vi "acquisition test fixed exposure 3.vi"() -> ()   [LabVIEW 2023]
uses:
  <vilib>/vision/driver/IMAQdx.llb/IMAQdx Attribute Type.ctl
  <vilib>/userDefined/High Color/IMAQdx.ctl
  <vilib>/vision/driver/IMAQdx.llb/IMAQdx Buffer Number Mode.ctl
  <vilib>/DAQmx/read.llb/DAQmx Read (Analog 1D Wfm NChan NSamp).vi
  <extravilib>/ChannelInstances/Tag-bool/Read With Abort.vi
  <extravilib>/ChannelInstances/Tag-bool/Write With Abort.vi
  <vilib>/DAQmx/create/channels.llb/DAQmx Create Channel (AI-Voltage-Basic).vi
  <vilib>/DAQmx/configure/timing.llb/DAQmx Timing (Sample Clock).vi
  <extravilib>/ChannelInstances/Tag-bool/Instantiate.vi
  <extravilib>/ChannelInstances/Tag-bool/EndpointRead.vi
  <extravilib>/ChannelInstances/Tag-bool/Endpoint.vi
  <vilib>/DAQmx/miscellaneous.llb/DAQmx Fill In Error Info.vi
  <extravilib>/ChannelInstances/Tag-bool.lvlib
  <vilib>/vision/driver/NI_Vision_Acquisition_Software.lvlib
  <resource>/objmgr/imaqdx.rc
panel:
  out "Maximum FrameRate":dbl
  out "Attribute Information":T2
  out "error out":errorcluster
  out "Sensor Readout Time":dbl
  out "Attribute Information Array 2":T3(array[cluster])
  out "Images Missed":u32
  out "Images Behind":i32
  out "Processed Frames per Second":dbl
  out "Acquired Frames per Second":dbl
  out "Image":T4(plugin-control)
  out "Waveform Chart":waveform(dbl)[](graph)
  in  "stop":bool
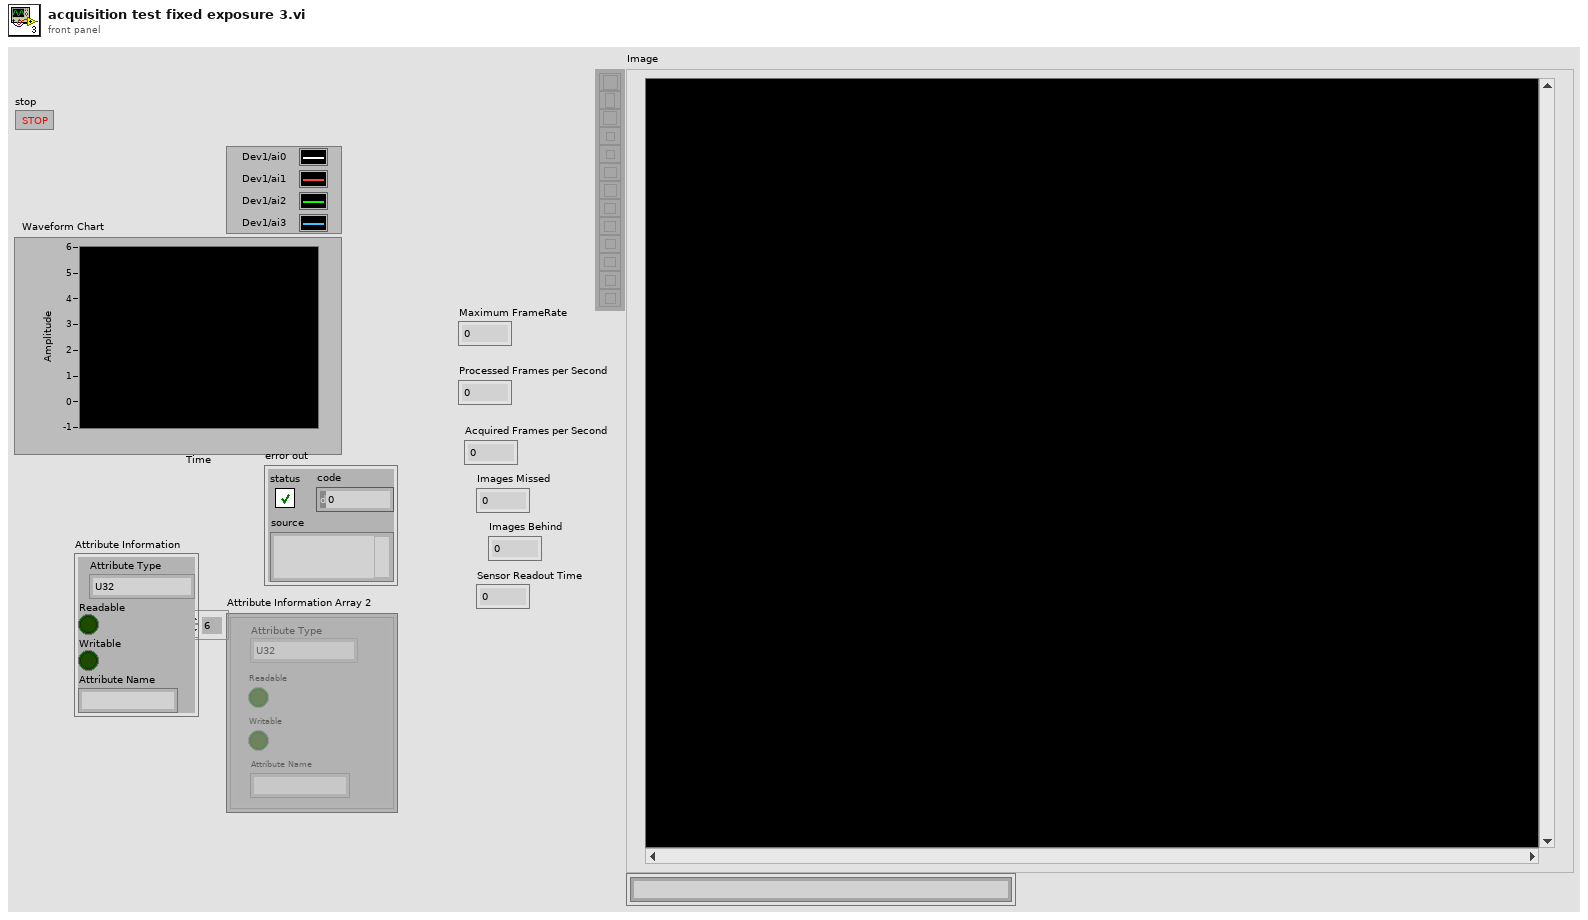
[diagram p1: front panel]
types:
  T1 = typedef "NI_Vision_Acquisition_Software.lvlib/IMAQdx Attribute Type.ctl" = enum32{"U32", "I64", "DBL", "String", "Enum", "Bool", "Command"}
  T2 = cluster{"Attribute Type":T1, "Readable":bool, "Writable":bool, "Attribute Name":string}
  T3 = cluster{"Attribute Type":T1, "Readable":bool, "Writable":bool, "Attribute Name":string}[]
  T4 = typedef "IMAQ Image.ctl" = refnum<image>
  T5 = enum16{"Exposure End", "Exposure Center", "Exposure Start", "Start", "NoSync"}
  T6 = typedef "IMAQdx.ctl" = refnum<k21>
  T7 = typedef "IMAQ AVI2 Refnum.ctl" = refnum<k20>
  T8 = typedef "Tag-bool.lvlib/))Channel.ctl" = refnum<queue>
  T9 = typedef "NI_Vision_Acquisition_Software.lvlib/IMAQdx Buffer Number Mode.ctl" = enum32{"Next", "Last", "Buffer Number", "Every", "Last New"}
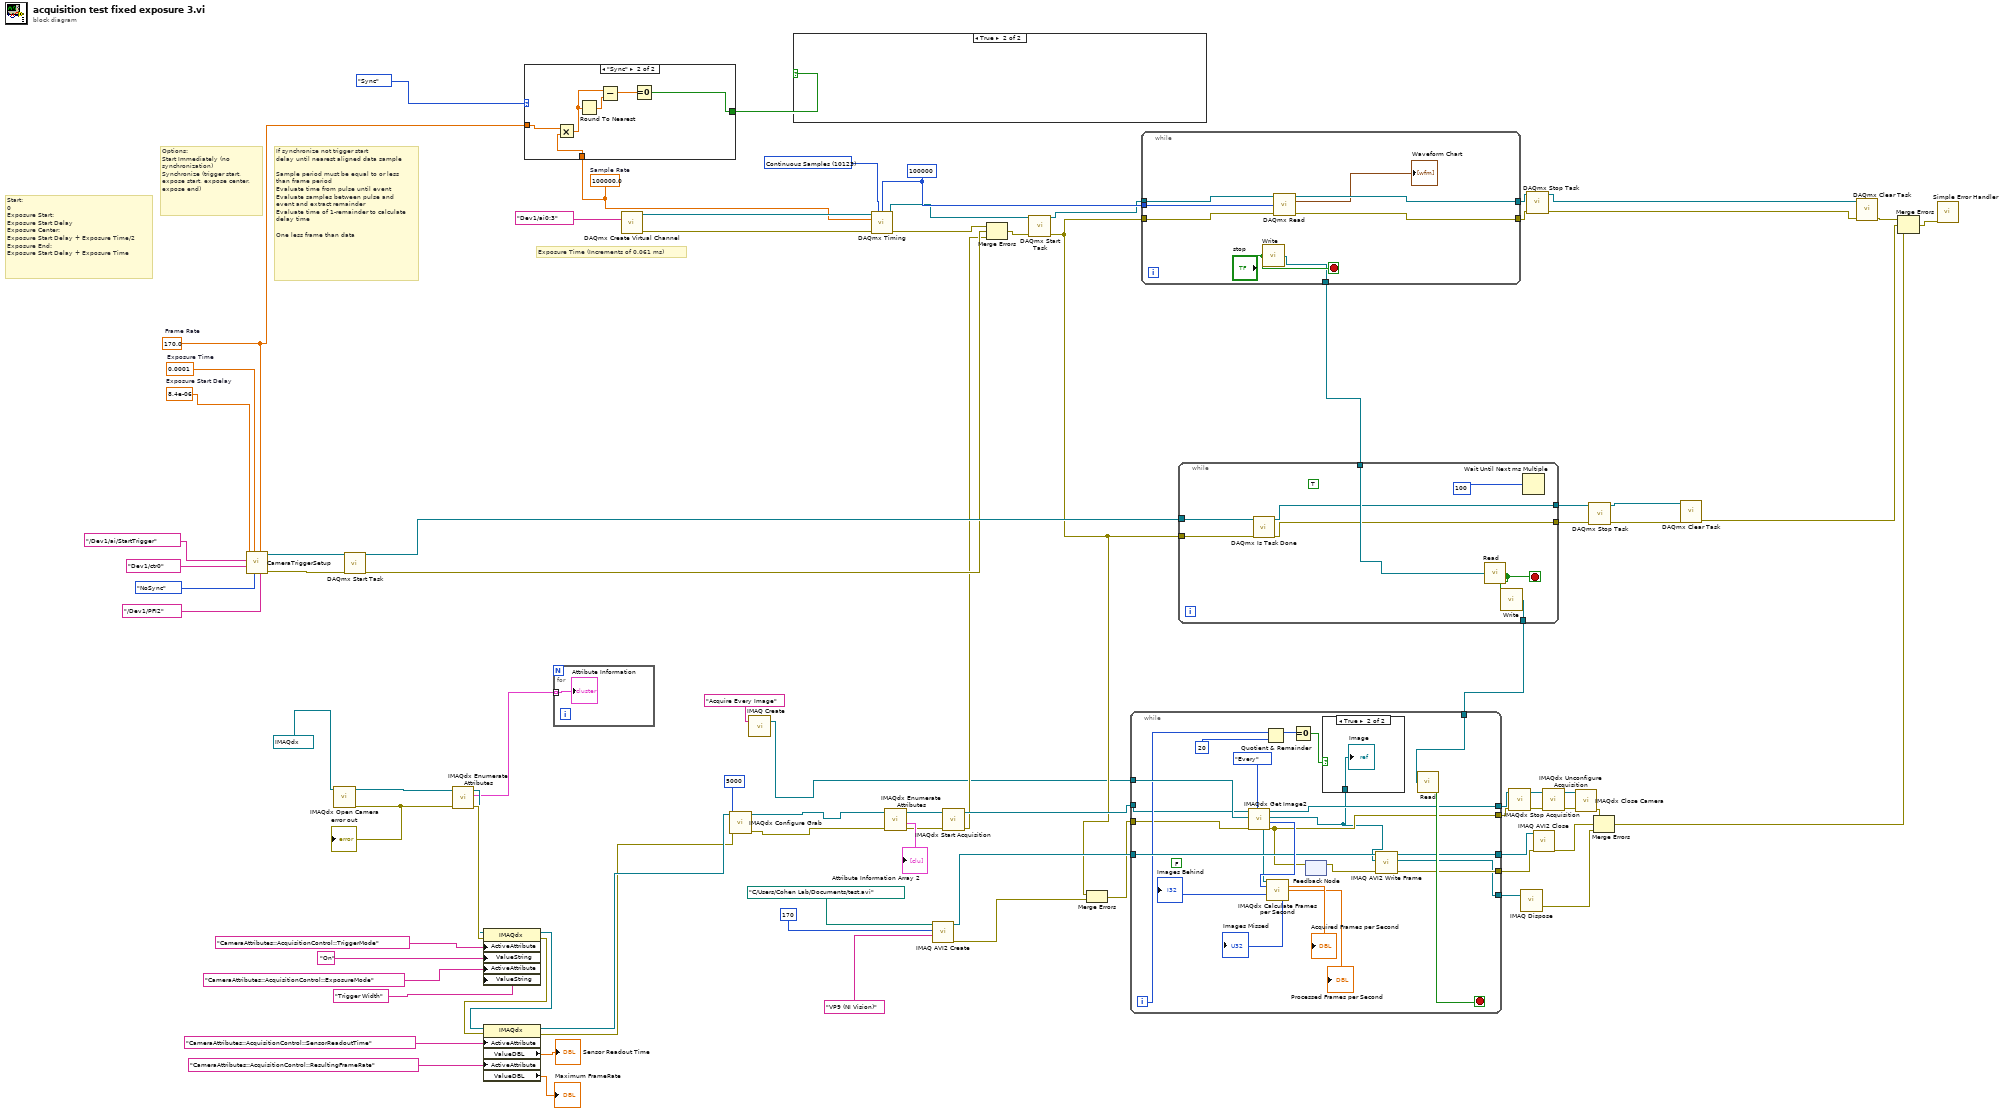
[diagram p0: block diagram]
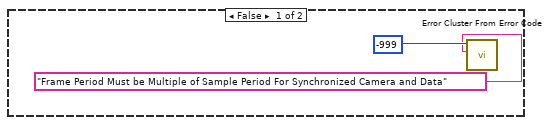
[diagram p2: hidden frame]
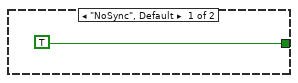
[diagram p3: hidden frame]
diagram:
  w46 = 8.4e-06  # Exposure Start Delay
  w42 = 170.0  # Frame Rate
  w45 = 0.0001  # Exposure Time
  w80 = 10123 items=["Finite Samples"=10178, "Continuous Samples"=10123, "Hardware Timed Single Point"=12522] ("sample mode")
  w81 = 100000 ("number of samples per channel")
  w43 = 100000.0  # Sample Rate
  # "Start:\n0\nExposure Start:\nExposure Start Delay\nExposure Center:\nExposure Start Delay + Exposure Time/2\nExposure End:\nExposure Start Delay + Exposure Time"
  # "If synchronize not trigger start\ndelay until nearest aligned data sample\n\nSample period must be equal to or less than frame period\nEvaluate time from pulse until event\nEvaluate samples between pulse and event and extract remainder\nEvaluate time of 1-remainder to calculate delay time\n\nOne less frame than data"
  # "Options:\nStart Immediately (no synchronization)\nSynchronize (trigger start, expose start, expose center, expose end)"
  # "Exposure Time (Increments of 0.061 ms)"
  n1 = call "CameraTriggerSetup.vi"("Camera\nTrigger\nOutput"=tag "/Dev1/PFI2" ("CO.Pulse.Term"), "Frame Rate"=w42, "Sync Type"=T5."NoSync", "Exposure Time"=w45, "Camera\nClock\nCounter"=tag "Dev1/ctr0" ("counter"), "Start Trigger Source"=tag "/Dev1/ai/StartTrigger" ("source"), "Exposure Start Delay"=w46) -> ("error out"=w39:errorcluster, "Refnum out"=w40:refnum<k21>)  [unwired: 3 in]
  n2 = call <vilib>:"IMAQdx Open Camera.vi"("Session In"=T6 "cam0") -> ("error out"=w64:errorcluster, "Session Out"=w72:T6)  [unwired: 9 in]
  "error out" <- w64
  n3 = call <vilib>:"DAQmx Start Task.vi"("task/channels in"=w40, "error in"=w39) -> ("task out"=w38:refnum<k21>, "error out"=w25:errorcluster)  [unwired: 12 in]
  n4 = call <vilib>:"IMAQdx Enumerate Attributes.vi"("error in"=w64, "Session In"=w72) -> ("error out"=w71:errorcluster, "Attribute Information Array"=w59:T3, "Session Out"=w70:T6)  [unwired: 7 in]
  n5 = property class="IMAQdx"(reference=w70, error in=w71, "ActiveAttribute"="CameraAttributes::AcquisitionControl::TriggerMode", "ValueString"="On", "ActiveAttribute"="CameraAttributes::AcquisitionControl::ExposureMode", "ValueString"="Trigger Width") -> (reference out=w61:T6, error out=w60:errorcluster)
  n6 = property class="IMAQdx"(reference=w61, error in=w60, "ActiveAttribute"="CameraAttributes::AcquisitionControl::SensorReadoutTime", "ActiveAttribute"="CameraAttributes::AcquisitionControl::ResultingFrameRate") -> (reference out=w68:T6, error out=w67:errorcluster, "ValueDBL"=→"Sensor Readout Time":dbl, "ValueDBL"=→"Maximum FrameRate":dbl)
  n7 = case shown="\"Sync\"" enum16{"NoSync", "Sync"}."Sync" {
    tunnel: [TRUE w86] -> w41
    tunnel: w42 -> [_ w91]
    tunnel: w43 -> [_ w90]
    frame "NoSync", Default {
    }
    frame "Sync" {
      n8 = Multiply(x=w91, y=w90) -> (x*y=w87:dbl)
      n9 = Round To Nearest(number=w87) -> (nearest integer value=w89:dbl)
      n10 = Subtract(x=w87, y=w89) -> (x-y=w88:dbl)
      n11 = Equal To 0?(x=w88) -> (x = 0?=w86:bool)
    }
  }
  n12 = for {
    tunnel: w59 -> [w92] mode=indexing
    "Attribute Information" <- w92
  }
  n13 = call-poly <vilib>:"DAQmx Create Virtual Channel.vi"("physical channels"=tag "Dev1/ai0:3") -> ("task out"=w84:refnum<k21>, "error out"=w83:errorcluster)  [unwired: 13 in]
  n14 = call <vilib>:"IMAQdx Configure Grab.vi"("error in"=w67, "Number of Buffers"=u32 5000, "Session In"=w68) -> ("error out"=w9:errorcluster, "Session Out"=w8:T6)  [unwired: 7 in]
  n15 = call "IMAQ Create"("Image Name"="Acquire Every Image") -> ("New Image"=w7:T4)  [unwired: 3 in, 2 out]
  n16 = case shown="True" w41 {
    frame False {
      n17 = call <vilib>:"Error Cluster From Error Code.vi"("error message (\"\")"="Frame Period Must be Multiple of Sample Period For Synchronized Camera and Data" ("source"), "error code (0)"=-999 ("code")) -> ()  [unwired: 7 in, 1 out]
    }
    frame True {
    }
  }
  n18 = call-poly <vilib>:"DAQmx Timing.vi"("task/channels in"=w84, "sample mode"=w80, "samples per channel"=w81, "rate"=w43, "error in"=w83) -> ("task out"=w37:refnum<k21>, "error out"=w32:errorcluster)  [unwired: 9 in]
  n19 = call <vilib>:"IMAQdx Enumerate Attributes.vi"("error in"=w9, "Session In"=w8) -> ("error out"=w35:errorcluster, "Attribute Information Array"=→"Attribute Information Array 2":T3, "Session Out"=w34:T6)  [unwired: 7 in]
  n20 = call "IMAQ AVI2 Create"("Codec"="VP9 (NI Vision)", "Frames Per Second"=u32 170, "AVI Path"=path "C:/Users/Cohen Lab/Documents/test.avi") -> ("error out"=w22:errorcluster, "AVI Refnum"=w27:T7)  [unwired: 7 in]
  n21 = call <vilib>:"IMAQdx Start Acquisition.vi"("error in"=w35, "Session In"=w34) -> ("error out"=w24:errorcluster, "Session Out"=w33:T6)  [unwired: 8 in]
  n22 = Merge Errors(w32, w25, w24) -> (w31:errorcluster)
  n23 = call <vilib>:"DAQmx Start Task.vi"("task/channels in"=w37, "error in"=w31) -> ("task out"=w36:refnum<k21>, "error out"=w23:errorcluster)  [unwired: 12 in]
  n24 = Merge Errors(w23, w22) -> (w21:errorcluster)
  n25 = while {
    tunnel: [w102] -> w57
    tunnel: [w101] -> w56
    tunnel: w36 -> [w100]
    tunnel: w23 -> [w99]
    tunnel: w81 -> [w98]
    tunnel: [w95] -> w79
    stop <- "stop" stop-if-true
    n26 = call <extravilib>:"Write.vi"("element"="stop") -> ("channel"=w95:T8)  [unwired: 1 out]
    n27 = call-poly <vilib>:"DAQmx Read.vi"("task/channels in"=w100, "number of samples per channel"=w98, "error in"=w99) -> ("task out"=w102:refnum<k21>, "data"=→"Waveform Chart":waveform(dbl)[], "error out"=w101:errorcluster)  [unwired: 10 in]
  }
  n28 = while {
    tunnel: w79 -> [w110]
    tunnel: [w108] -> w78
    tunnel: w38 -> [w107]
    tunnel: w23 -> [w106]
    tunnel: [w105] -> w53
    tunnel: [w104] -> w52
    stop <- w109 stop-if-true
    (unwired) TRUE ("auto start")
    n29 = call <vilib>:"DAQmx Is Task Done.vi"("task/channels in"=w107, "error in"=w106) -> ("task out"=w105:refnum<k21>, "error out"=w104:errorcluster)  [unwired: 11 in, 1 out]
    n30 = call <extravilib>:"Read.vi"("channel"=w110) -> ("element"=w109:bool)  [unwired: 1 in, 1 out]
    n31 = call <extravilib>:"Write.vi"("element"=w109) -> ("channel"=w108:T8)  [unwired: 1 out]
    n32 = Wait Until Next ms Multiple(millisecond multiple=u32 100) -> ()  [unwired: 1 out]
  }
  n33 = while {
    tunnel: w78 -> [w133]
    tunnel: w33 -> [w117]
    tunnel: w21 -> [w116]
    tunnel: [w113] -> w4
    tunnel: w7 -> [w131]
    tunnel: w27 -> [w125]
    tunnel: [w124] -> w26
    tunnel: [w123] -> w20
    tunnel: [w122] -> w11
    tunnel: [w112] -> w2
    i -> [w119]
    stop <- w132 stop-if-true
    (unwired) FALSE ("Release Previous (true)")
    n34 = call <vilib>:"IMAQdx Get Image2.vi"("Buffer Number Mode (Next)"=IMAQdx_Buffer_Number_Mode."Every", "error in"=w116, "Image In"=w131, "Session In"=w117) -> ("error out"=w112:errorcluster, "Buffer Number Out"=w130:u32, "Image Out"=w111:T4, "Session Out"=w113:T6)  [unwired: 4 in]
    n35 = Quotient & Remainder(x=w119, y=20) -> (x-y*floor(x/y)=w121:i32)  [unwired: 1 out]
    n36 = call <vilib>:"IMAQdx Calculate Frames per Second.vi"("Session In"=w113, "Buffer Number"=w130) -> ("Acquired Frames per Second"=→"Acquired Frames per Second":dbl, "Processed Frames per Second"=→"Processed Frames per Second":dbl, "Images Behind"=→"Images Behind":i32, "Images Missed"=→"Images Missed":u32)  [unwired: 7 in, 3 out]
    n37 = Equal To 0?(x=w121) -> (x = 0?=w120:bool)
    n38 = feedback-in #1(w112) -> ()
    n39 = feedback #1() -> (w114:errorcluster)  [unwired: 1 in]
    n40 = case shown="True" w120 {
      tunnel: w111 -> [_ w134]
      frame False {
      }
      frame True {
        "Image" <- w134
      }
    }
    n41 = call "IMAQ AVI2 Write Frame"("error in (no error)"=w114, "Image"=w111, "AVI Refnum"=w125) -> ("error out"=w123:errorcluster, "Image Out (duplicate)"=w122:T4, "AVI Refnum (duplicate)"=w124:T7)  [unwired: 6 in]
    n42 = call <extravilib>:"Read.vi"("channel"=w133) -> ("element"=w132:bool)  [unwired: 1 in, 1 out]
  }
  n43 = call <vilib>:"IMAQdx Stop Acquisition.vi"("error in"=w2, "Session In"=w4) -> ("error out"=w5:errorcluster, "Session Out"=w6:T6)  [unwired: 8 out]
  n44 = call "IMAQ Dispose"("Image"=w11) -> ("error out"=w10:errorcluster)  [unwired: 5 in]
  n45 = call <vilib>:"DAQmx Stop Task.vi"("task/channels in"=w57, "error in"=w56) -> ("task out"=w55:refnum<k21>, "error out"=w17:errorcluster)  [unwired: 12 in]
  n46 = call "IMAQ AVI2 Close"("error in (no error)"=w20, "AVI Refnum"=w26) -> ("error out"=w18:errorcluster)  [unwired: 9 in]
  n47 = call <vilib>:"IMAQdx Unconfigure Acquisition.vi"("error in"=w5, "Session In"=w6) -> ("error out"=w3:errorcluster, "Session Out"=w1:T6)  [unwired: 8 out]
  n48 = call <vilib>:"IMAQdx Close Camera.vi"("error in"=w3, "Session In"=w1) -> ("error out"=w19:errorcluster)  [unwired: 9 in]
  n49 = call <vilib>:"DAQmx Stop Task.vi"("task/channels in"=w53, "error in"=w52) -> ("task out"=w58:refnum<k21>, "error out"=w16:errorcluster)  [unwired: 12 in]
  n50 = Merge Errors(w19, w18, w10) -> (w13:errorcluster)
  n51 = call <vilib>:"DAQmx Clear Task.vi"("task in"=w58, "error in"=w16) -> ("error out"=w14:errorcluster)  [unwired: 13 in]
  n52 = call <vilib>:"DAQmx Clear Task.vi"("task in"=w55, "error in"=w17) -> ("error out"=w15:errorcluster)  [unwired: 13 in]
  n53 = Merge Errors(w15, w14, w13) -> (w12:errorcluster)
  n54 = call <vilib>:"Simple Error Handler.vi"("error in (no error)"=w12) -> ()  [unwired: 4 in, 5 out]
